vi "Add Alias_Alias Internal.vi"(8 "error in (no error)":errorcluster, 10 "Name":string, 11 "Base Node":refnum<k24>) -> (0 "error out":errorcluster, 3 "Base Node out":refnum<k24>)   [LabVIEW 2019, in "Simple SysDef API.lvlib"]
uses:
  <userlib>/SimpleSysDef/Simple SysDef API.lvlib
  NationalInstruments.VeriStand.SystemDefinitionAPI
  <userlib>/SimpleSysDef/_SubVIs/Add Alias_Alias Settings.ctl
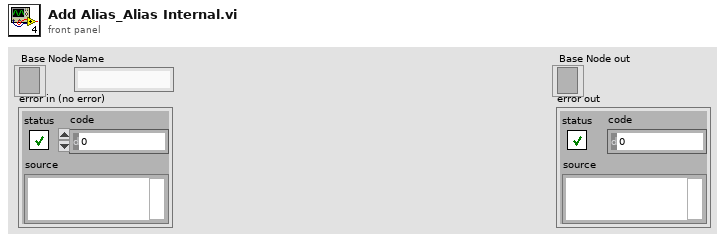
[diagram p1: front panel]
types:
  T1 = typedef "Simple SysDef API.lvlib/Add Alias_Alias Settings.ctl" = cluster{"Name":string, "Description":string, "LinkedChannelPath":string}
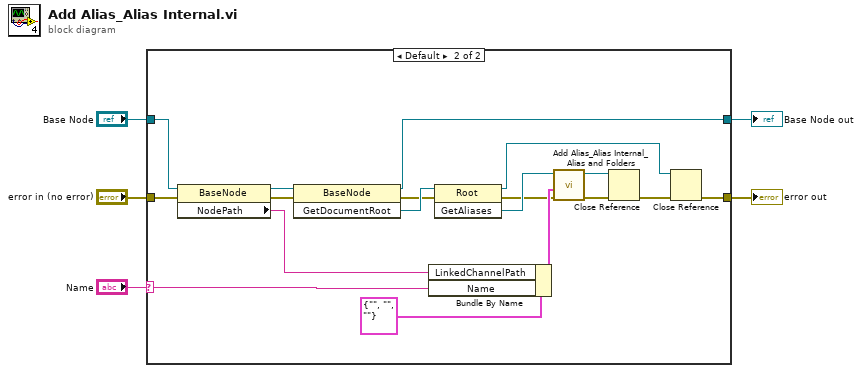
[diagram p0: block diagram]
diagram:
  n1 = case shown="Default" "Name" {
    selector: "Name" -> [_ w23]
    tunnel: [w7 w18] -> w5
    tunnel: [w6 w14] -> w4
    tunnel: "error in (no error)" -> [w6 w25]
    tunnel: "Base Node" -> [w7 w24]
    frame "" {
    }
    frame Default {
      n2 = property class="BaseNode"(reference=w24, error in=w25) -> (reference out=w19:refnum<k24>, error out=w20:errorcluster, "NodePath"=w21:string)
      n3 = invoke class="BaseNode" method="GetDocumentRoot"(reference=w19, error in=w20) -> (reference out=w18:refnum<k24>, error out=w16:errorcluster, "GetDocumentRoot"=w17:refnum<k24>)  [unwired: 1 in]
      n4 = Bundle By Name(cluster=T1 {"Name"="", "Description"="", "LinkedChannelPath"=""} ("Alias Settings"), "LinkedChannelPath"=w21, "Name"=w23) -> (w11:T1)
      n5 = invoke class="Root" method="GetAliases"(reference=w17, error in=w16) -> (reference out=w13:refnum<k24>, error out=w10:errorcluster, "GetAliases"=w12:refnum<k24>)  [unwired: 1 in]
      n6 = call <userlib>:"Add Alias_Alias Internal_Alias and Folders.vi"("error in (no error)"=w10, "Alias Settings"=w11, "Alias Ref"=w12) -> ("error out"=w9:errorcluster, "Alias Ref Out"=w8:refnum<k24>)  [unwired: 7 in]
      n7 = Close Reference(reference=w8, error in (no error)=w9) -> (error out=w15:errorcluster)
      n8 = Close Reference(reference=w13, error in (no error)=w15) -> (error out=w14:errorcluster)
    }
  }
  "Base Node out" <- w5
  "error out" <- w4
